vi "TBA_NET_Close.vi"(8 "error in (no error)":errorcluster caption="错误输入（无错误）", 11 "ToolStrip 输入":refnum<class "ToolStrip.lvclass"> caption="Toolbar Ref") -> (0 "error out":errorcluster caption="错误输出")   [LabVIEW 2016, in "ToolStrip.lvclass"]
uses:
  Pravite/ToolStrip.lvclass
  Pravite/ToolStrip.lvclass/ToolStrip.ctl
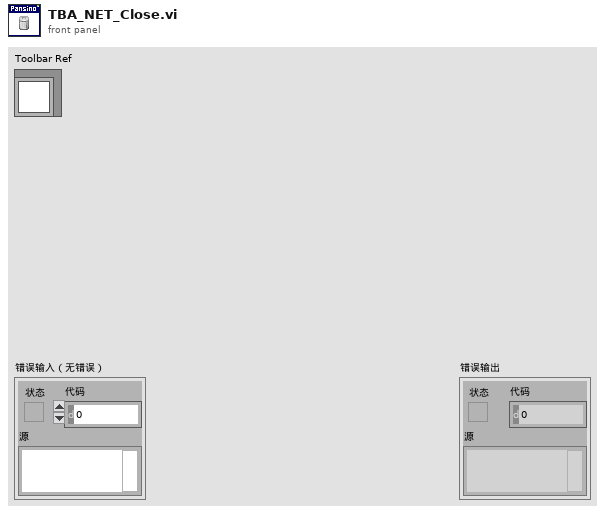
[diagram p1: front panel]
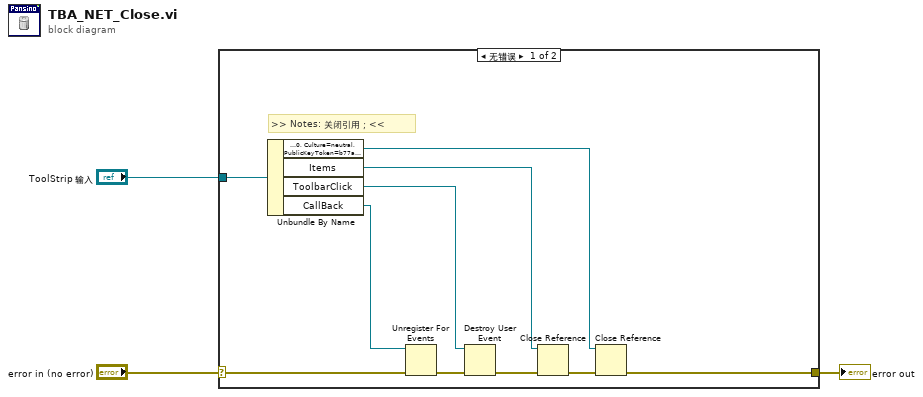
[diagram p0: block diagram]
diagram:
  n1 = case shown="无错误" "error in (no error)" {
    selector: "error in (no error)" -> [w5 w14]
    tunnel: [w4 w14] -> w2
    tunnel: "ToolStrip 输入" -> [w13 _]
    frame No Error {
      # ">> Notes: 关闭引用；<<"
      n2 = Unbundle By Name(w13) -> ("ToolStrip"=w6:refnum<k24>, "Items"=w7:refnum<k24>, "ToolbarClick"=w8:refnum<user-event>, "CallBack"=w9:refnum<k27>)
      n3 = Unregister For Events(event registration refnum=w9, error in=w5) -> (error out=w11:errorcluster)
      n4 = Destroy User Event(user event=w8, error in=w11) -> (error out=w10:errorcluster)
      n5 = Close Reference(reference=w7, error in (no error)=w10) -> (error out=w12:errorcluster)
      n6 = Close Reference(reference=w6, error in (no error)=w12) -> (error out=w4:errorcluster)
    }
    frame Error {
    }
  }
  "error out" <- w2
